vi "StreamChansValid.vi"(0 "BitMaskRequested":bool[](array[boolean]), 11 "MaxStreamChans":u16) -> (1 "bitMaskModified":bool[](array[boolean]), 2 "NumRequested":i16, 3 "AccelList":u16[](array[numeric]), 4 "AmpsList":u16[](array[numeric]), 10 "VddList":u16[](array[numeric]), 12 "bitMaskI16":i16[](array[numeric]), 15 "NumStreamingCluster":T1)   [LabVIEW 2020]
doc: "Takes as input binary bitmask for streaming channels and the max number of channels that can be streamed.\n\nOutputs the bitmask subset corresponding to the first N chans, if Nrequested > Nmax channels that can be streamed.\n\nNumChansStreaming is the total number of channels that are streaming (amps + accel + vbat)\n\nbitMaskI16 is the numeric representation (0,1) of the boolean array bitMaskModified that specifies which channels are actually streaming.\n\nStreamChanList is an array of integer numbers specifying which channels are streaming (0-127 for amps A-D) + 128-130 (ax,ay,az) + 131 Vbat"
panel:
  out "VflexList":u16[](array[numeric])
  out "NumChansStreaming":i16
  out "finalarrysz":i32
  out "leftoverelements":i32
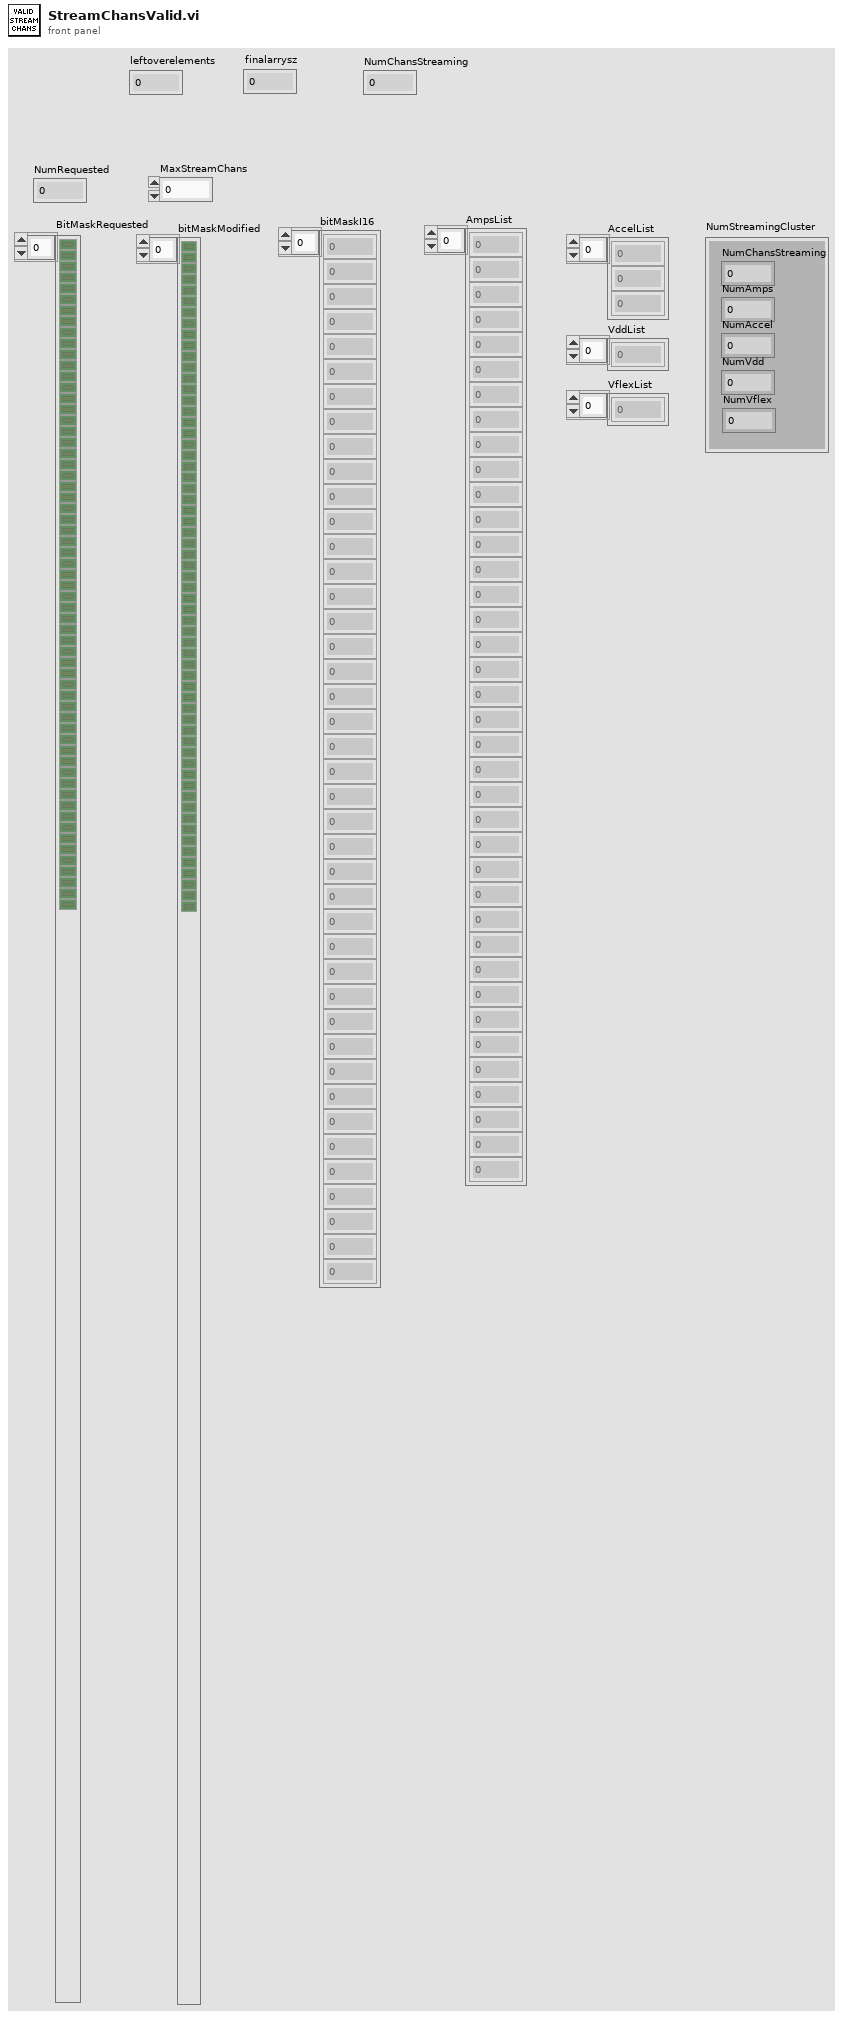
[diagram p1: front panel]
types:
  T1 = cluster{"NumChansStreaming":i16, "NumAmps":i32, "NumAccel":i32, "NumVdd":i32, "NumVflex":i32}
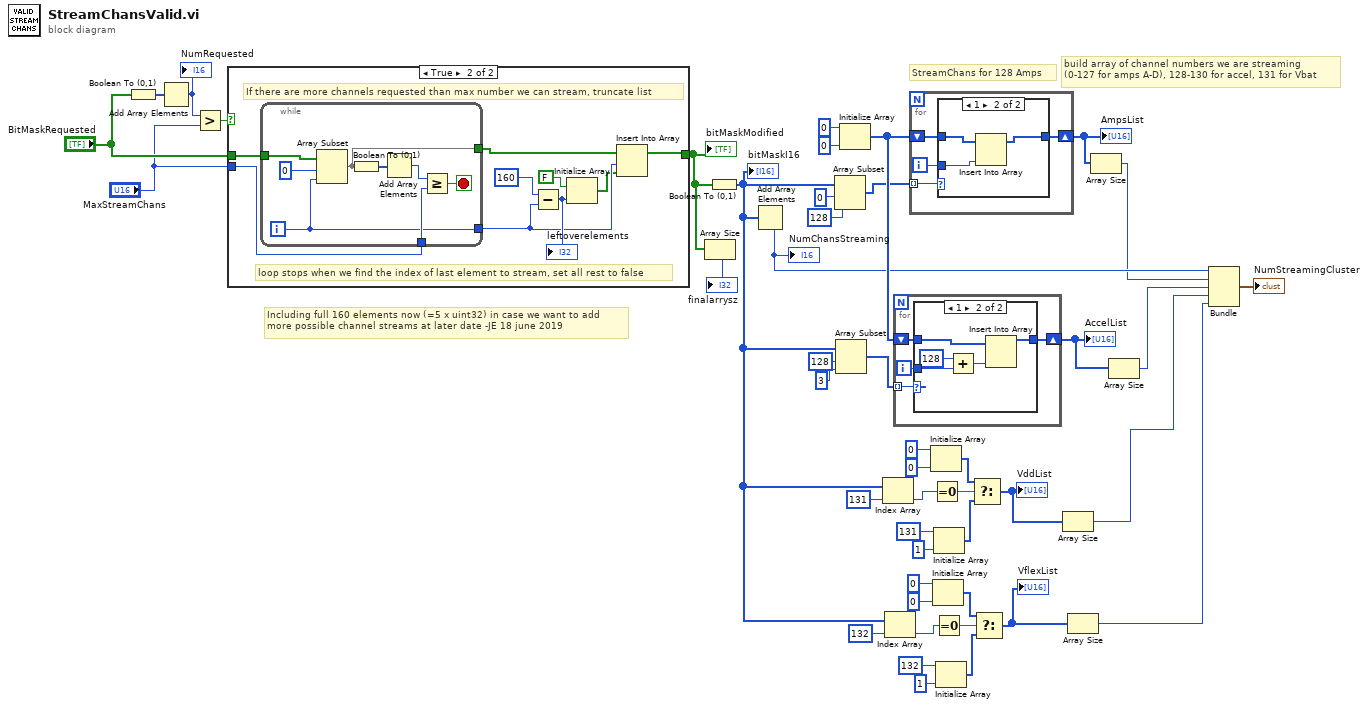
[diagram p0: block diagram]
diagram:
  # "StreamChans for 128 Amps"
  # "Including full 160 elements now (=5 x uint32) in case we want to add\nmore possible channel streams at later date -JE 18 june 2019"
  # "build array of channel numbers we are streaming\n(0-127 for amps A-D), 128-130 for accel, 131 for Vbat"
  n1 = Boolean To (0,1)(Boolean="BitMaskRequested") -> (0, 1=w44:i16[])
  n2 = Add Array Elements(numeric array=w44) -> (sum=w43:i16)
  "NumRequested" <- w43
  n3 = Greater?(x=w43, y="MaxStreamChans") -> (0:w41:bool)
  n4 = case shown="True" w41 {
    tunnel: "MaxStreamChans" -> [_ w54]
    tunnel: [w46 w48] -> w38
    tunnel: "BitMaskRequested" -> [w46 w55]
    frame False {
      # "nothing to modify"
    }
    frame True {
      # "If there are more channels requested than max number we can stream, truncate list"
      # "loop stops when we find the index of last element to stream, set all rest to false"
      n5 = while {
        tunnel: w55 -> [w63]
        tunnel: w54 -> [w60]
        tunnel: [w56] -> w50
        tunnel: [w58] -> w53
        i -> [w56]
        stop <- w59 stop-if-true
        n6 = Array Subset(array=w63, index=0, length=w56) -> (w58:bool[])
        n7 = Boolean To (0,1)(Boolean=w58) -> (0, 1=w62:i16[])
        n8 = Add Array Elements(numeric array=w62) -> (sum=w61:i16)
        n9 = Greater Or Equal?(x=w61, y=w60) -> (x >= y?=w59:bool)
      }
      n10 = Subtract(x=160, y=w50) -> (x-y=w51:i32)
      "leftoverelements" <- w51
      n11 = Initialize Array(FALSE, w51) -> (w49:bool[])
      n12 = Insert Into Array(array=w53, index=w50, new element=w49) -> (w48:bool[])
    }
  }
  "bitMaskModified" <- w38
  n13 = Array Size(array=w38) -> (size(s)=→"finalarrysz":i32)
  n14 = Boolean To (0,1)(Boolean=w38) -> (0, 1=w2:i16[])
  "bitMaskI16" <- w2
  n15 = Add Array Elements(numeric array=w2) -> (sum=w17:i16)
  "NumChansStreaming" <- w17
  n16 = Array Subset(array=w2, index=0, length=128) -> (w35:i16[])
  n17 = Array Subset(array=w2, index=128, length=3 ("index")) -> (w30:i16[])
  n18 = Initialize Array(u16 0 ("element"), 0 ("dimension size")) -> (w36:u16[])
  n19 = Index Array(array=w2, index=131) -> (element=w28:i16)
  n20 = Index Array(array=w2, index=132) -> (element=w1:i16)
  n21 = for {
    tunnel: w30 -> [w67] mode=indexing
    shift-right: [w64] -> w19
    shift-left: w36 -> [w65]
    i -> [w66]
    n22 = case shown="1" w67 {
      tunnel: w66 -> [_ w73]
      tunnel: w65 -> [w68 w72]
      tunnel: [w68 w71] -> w64
      frame 0, Default {
      }
      frame 1 {
        n23 = Add(x=128, y=w73) -> (x+y=w70:i32)
        n24 = Insert Into Array(array=w72, new element=w70) -> (w71:u16[])  [unwired: 1 in]
      }
    }
  }
  "AccelList" <- w19
  n25 = for {
    tunnel: w35 -> [w77] mode=indexing
    shift-right: [w74] -> w20
    shift-left: w36 -> [w75]
    i -> [w76]
    n26 = case shown="1" w77 {
      tunnel: w76 -> [_ w81]
      tunnel: w75 -> [w78 w80]
      tunnel: [w78 w79] -> w74
      frame 0, Default {
      }
      frame 1 {
        n27 = Insert Into Array(array=w80, new element=w81) -> (w79:u16[])  [unwired: 1 in]
      }
    }
  }
  "AmpsList" <- w20
  n28 = Initialize Array(u16 0 ("element"), 0 ("dimension size")) -> (w24:u16[])
  n29 = Equal To 0?(x=w28) -> (x = 0?=w27:bool)
  n30 = Initialize Array(u16 0 ("element"), 0 ("dimension size")) -> (w7:u16[])
  n31 = Initialize Array(u16 131 ("element"), 1 ("dimension size")) -> (w21:u16[])
  n32 = Equal To 0?(x=w1) -> (x = 0?=w10:bool)
  n33 = Initialize Array(u16 132 ("element"), 1 ("dimension size")) -> (w4:u16[])
  n34 = Select(t=w24, s=w27, f=w21) -> (s? t:f=w18:u16[])
  "VddList" <- w18
  n35 = Select(t=w7, s=w10, f=w4) -> (s? t:f=w3:u16[])
  "VflexList" <- w3
  n36 = Array Size(array=w18) -> (size(s)=w13:i32)
  n37 = Array Size(array=w3) -> (size(s)=w12:i32)
  n38 = Array Size(array=w20) -> (size(s)=w15:i32)
  n39 = Array Size(array=w19) -> (size(s)=w14:i32)
  n40 = Bundle("Boolean"=w17, w15, w14, w13, w12) -> (→"NumStreamingCluster":cluster{"Boolean":i16, i32, i32, i32, i32})  [unwired: 1 in]
